vi "ConvertTdmsFileToNoDaqMxRaw_2011.vi"(6 "Error In":errorcluster, 7 "File conver to":path, 8 "File convert from":path) -> (0 "Error Out":errorcluster)   [LabVIEW 2013]
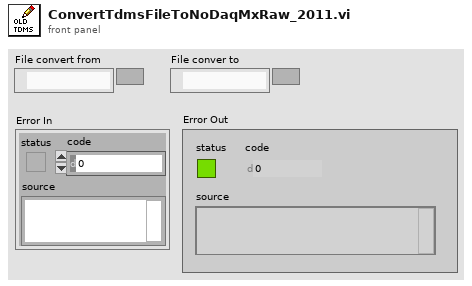
[diagram p1: front panel]
types:
  T1 = enum16{"open", "open or create", "create or replace", "create", "open (read-only)"}
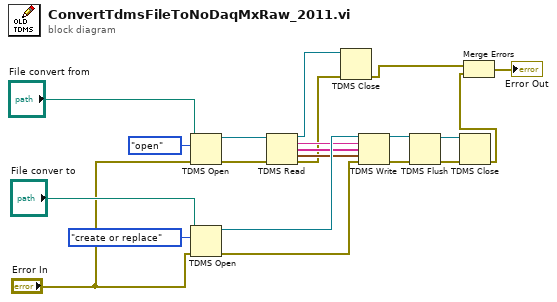
[diagram p0: block diagram]
diagram:
  n1 = TDMS Open(8:"Error In", 10:T1."open" ("operation (0:open)"), 11:"File convert from") -> (0:w6:errorcluster, 3:w5:refnum<k34>)  [unwired: 4 in]
  n2 = TDMS Open(8:"Error In", 10:T1."create or replace" ("operation (0:open)"), 11:"File conver to") -> (0:w12:errorcluster, 3:w13:refnum<k34>)  [unwired: 4 in]
  n3 = TDMS Read(0:w5, 11:w6) -> (4:w8:refnum<k34>, 6:w9:string, 8:w10:string[], 10:w11:waveform(dbl)[], 15:w7:errorcluster)  [unwired: 6 in, 1 out]
  n4 = TDMS Close(8:w7, 11:w8) -> (0:w21:errorcluster)  [unwired: 1 out]
  n5 = TDMS Write(0:w13, 5:w9, 7:w10, 9:w11, 11:w12) -> (4:w14:refnum<k34>, 15:w15:errorcluster)  [unwired: 1 in, 2 out]
  n6 = TDMS Flush(4:w15, 7:w14) -> (0:w19:errorcluster, 3:w18:refnum<k34>)
  n7 = TDMS Close(8:w19, 11:w18) -> (0:w20:errorcluster)  [unwired: 1 out]
  n8 = Merge Errors(w21, w20) -> (→"Error Out":errorcluster)
